vi "Set Multi Track Scan.vi"(0 "trackHeight":i32, 1 "trackHBinning":i32, 2 "trackGap":i32, 3 "trackSkip":i32, 5 "numberTracks":i32, 7 "iSIHStart":i32, 9 "iSIHEnd":i32, 11 "error in (no error)":errorcluster, 12 "trackVBinning":i32, 13 "trackOffset":i32, 14 "numberSubFrames":i32) -> (4 "function return":u32, 15 "error out":errorcluster)   [LabVIEW 2014, in "atmcd32d.lvlib"]
doc: "unsigned int WINAPI SetMultiTrackScan(int trackHeight, int numberTracks, int iSIHStart, int iSIHEnd, int trackHBinning, int trackVBinning, int trackGap, int trackOffset, int trackSkip, int numberSubFrames);"
uses:
  atmcd32d.lvlib
  atmcd32d.dll
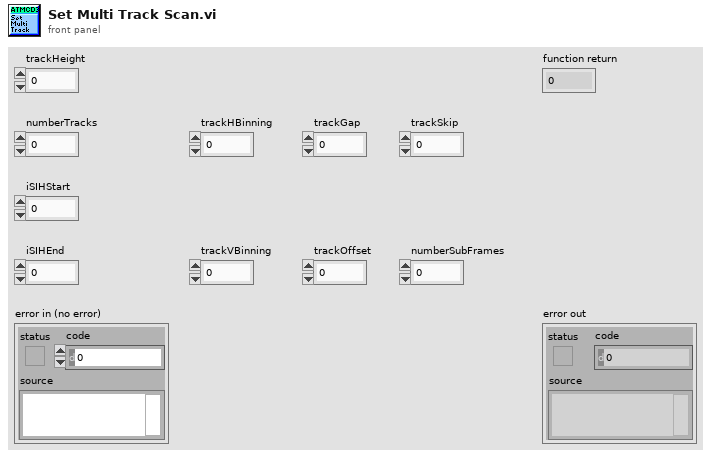
[diagram p1: front panel]
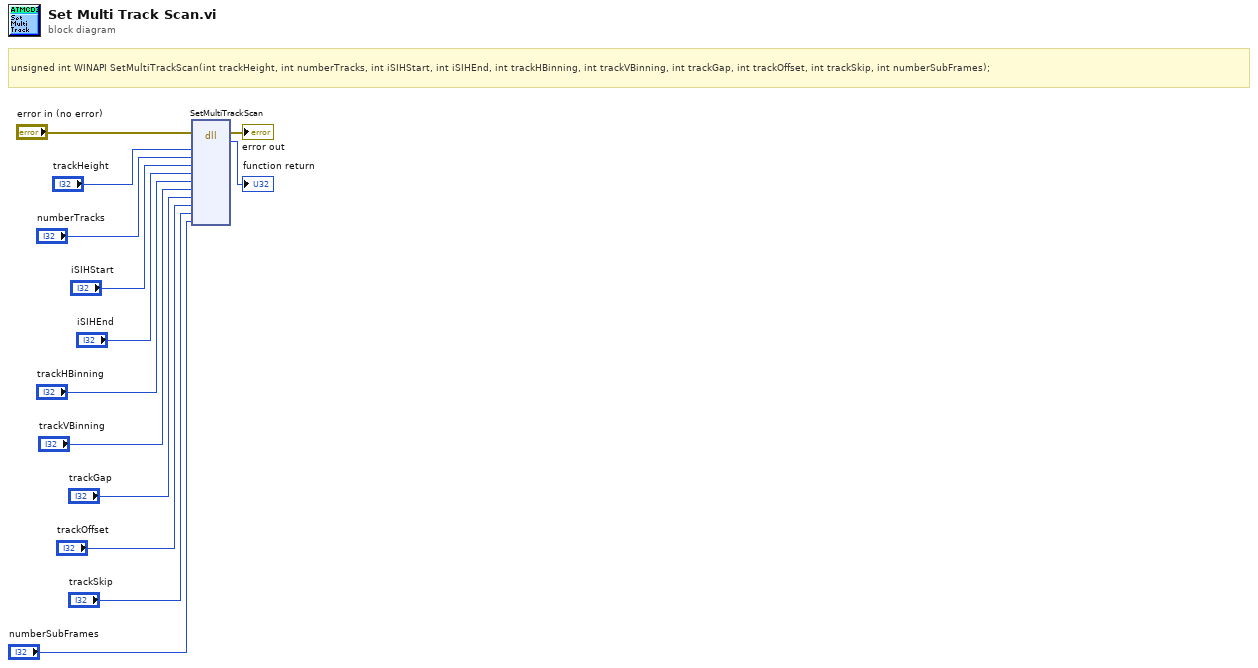
[diagram p0: block diagram]
diagram:
  # "unsigned int WINAPI SetMultiTrackScan(int trackHeight, int numberTracks, int iSIHStart, int iSIHEnd, int trackHBinning, int trackVBinning, int trackGap, int trackOffset, int trackSkip, int numberSubFrames);"
  n1 = dll-call lib="C:/Users/Bakir/Documents/Lambda2-Testing/lib/Andorlib/atmcd32d.*" fn="SetMultiTrackScan"(error in="error in (no error)", "trackHeight"="trackHeight", "numberTracks"="numberTracks", "iSIHStart"="iSIHStart", "iSIHEnd"="iSIHEnd", "trackHBinning"="trackHBinning", "trackVBinning"="trackVBinning", "trackGap"="trackGap", "trackOffset"="trackOffset", "trackSkip"="trackSkip", "numberSubFrames"="numberSubFrames") -> (error out=→"error out":errorcluster, →"function return":u32)  [unwired: 12 in, 1 out]
